vi "Get Steering Frame Velocity from Single Wheel.vi"(4 "acquired wheel states":T2[](array[typedef]), 6 "get motor data":bool, 7 "index info":T1, 8 "error in (no error)":errorcluster, 9 "velocity transform vector in":dbl[](array[numeric]), 10 "velocity transform matrix in":T3, 11 "steering frame in":refnum<class "NI_Robotics_Steering Frame.lvclass">) -> (0 "error out":errorcluster, 1 "velocity transform vector out":dbl[](array[numeric]), 2 "velocity transform matrix out":T3, 3 "steering frame out":refnum<class "NI_Robotics_Steering Frame.lvclass">)   [LabVIEW 2017, in "NI_Robotics_Steering Frame.lvclass"]
uses:
  <vilib>/robotics/Steering/Steering Frame/NI_Robotics_Steering Frame.lvclass
  <vilib>/Analysis/Matrix/Datatypes/RealMatrix.ctl
  <vilib>/robotics/Steering/Wheel/Wheel State.ctl
  <vilib>/robotics/Steering/Steering Frame/NI_Robotics_Steering Frame.lvclass/NI_Robotics_Steering Frame.ctl
  <vilib>/robotics/Steering/Wheel/NI_Robotics_Wheel.lvclass
  <vilib>/Analysis/Matrix/NI_Matrix.lvlib
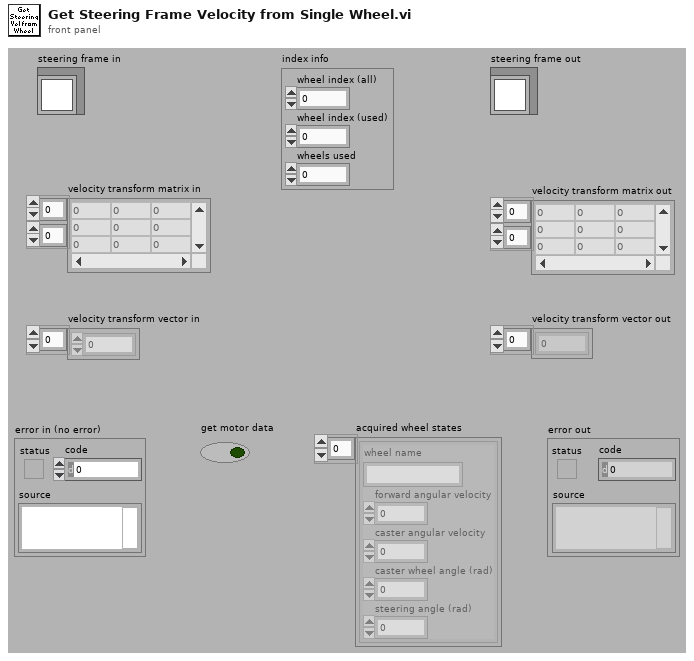
[diagram p1: front panel]
types:
  T1 = cluster{"wheel index (all)":i32, "wheel index (used)":i32, "wheels used":i32}
  T2 = typedef "NI_Robotics_Wheel.lvclass/Wheel State.ctl" = cluster{"wheel name":string, "forward angular velocity":dbl, "caster angular velocity":dbl, "caster wheel angle (rad)":dbl, "steering angle (rad)":dbl}
  T3 = typedef "NI_Matrix.lvlib/RealMatrix.ctl" = dbl[][]
  T4 = typedef "NI_Robotics_Steering Frame.lvclass/Wheel Orientation.ctl" = cluster{"wheel":refnum<class "NI_Robotics_Wheel.lvclass">, "x position":dbl, "y position":dbl, "frame angle (rad)":dbl}
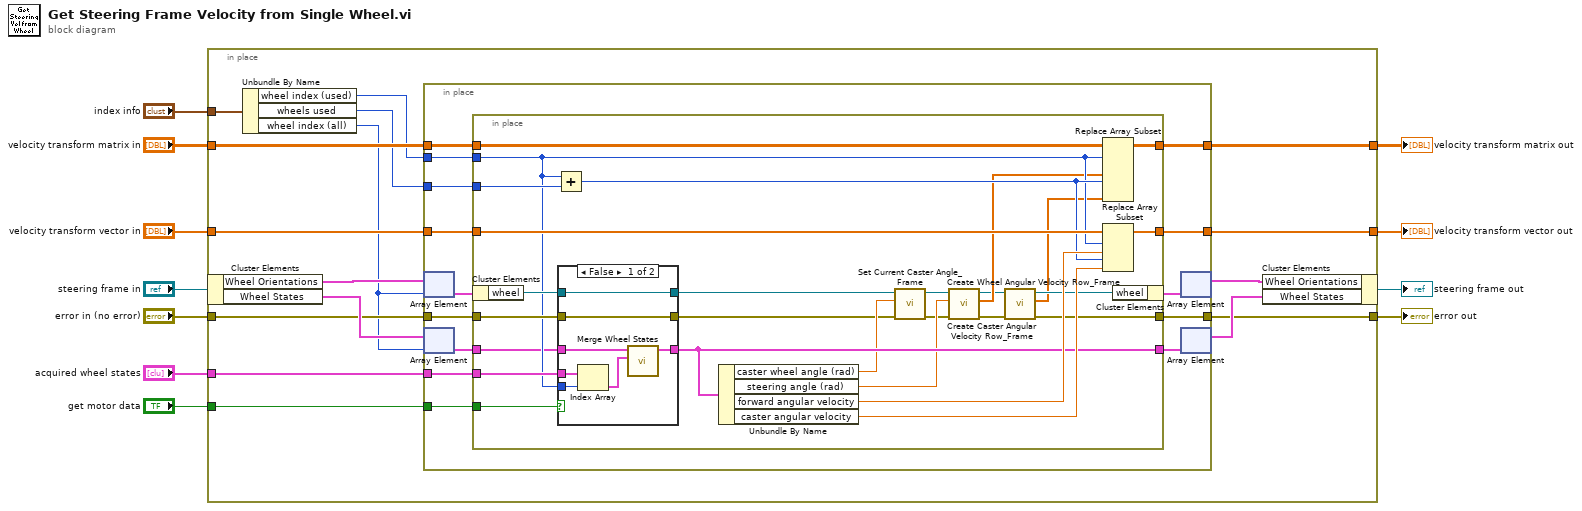
[diagram p0: block diagram]
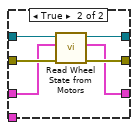
[diagram p2: hidden frame]
diagram:
  n1 = in-place {
    in-place-border: "error in (no error)" -> [w23]
    in-place-border: [w22] -> w8
    in-place-border: "velocity transform matrix in" -> [w21]
    in-place-border: "velocity transform vector in" -> [w20]
    in-place-border: "get motor data" -> [w19]
    in-place-border: "acquired wheel states" -> [w18]
    in-place-border: [w17] -> w3
    in-place-border: [w16] -> w2
    in-place-border: "index info" -> [w15]
    n2 = in-place-cluster #1("steering frame in") -> ("Wheel Orientations"=w27:T4[], "Wheel States"=w25:T2[])
    n3 = Unbundle By Name(w15) -> ("wheel index (used)"=w14:i32, "wheels used"=w13:i32, "wheel index (all)"=w12:i32)
    n4 = in-place {
      in-place-border: [w41] -> w22
      in-place-border: w23 -> [w40]
      in-place-border: w19 -> [w39]
      in-place-border: w20 -> [w38]
      in-place-border: [w37] -> w16
      in-place-border: w21 -> [w36]
      in-place-border: [w35] -> w17
      in-place-border: w13 -> [w34]
      in-place-border: w14 -> [w33]
      in-place-border: w18 -> [w32]
      n5 = in-place-array #2(w27, w12) -> (w31:T4)
      n6 = in-place-array #3(w25, w12) -> (w29:T2)
      n7 = in-place {
        in-place-border: [w47] -> w41
        in-place-border: w40 -> [w67]
        in-place-border: w29 -> [w55]
        in-place-border: w39 -> [w58]
        in-place-border: [w54] -> w28
        in-place-border: w38 -> [w66]
        in-place-border: [w65] -> w37
        in-place-border: w36 -> [w62]
        in-place-border: [w61] -> w35
        in-place-border: w34 -> [w60]
        in-place-border: w33 -> [w56]
        in-place-border: w32 -> [w57]
        n8 = in-place-cluster #4(w31) -> ("wheel"=w68:refnum<class "NI_Robotics_Wheel.lvclass">)
        n9 = Add(x=w56, y=w60) -> (x+y=w59:i32)
        n10 = case shown="False" w58 {
          tunnel: w68 -> [w75 w81]
          tunnel: w67 -> [w73 w80]
          tunnel: [w73 w79] -> w42
          tunnel: [w75 w78] -> w45
          tunnel: [w72 w77] -> w54
          tunnel: w55 -> [w74 w76]
          tunnel: w57 -> [w71 _]
          tunnel: w56 -> [w69 _]
          frame False {
            n11 = Index Array(array=w71, index=w69) -> (element=w70:T2)
            n12 = call <vilib>:"Merge Wheel States.vi"("wheel state with data"=w70, "wheel state with name"=w74) -> ("merged wheel state"=w72:T2)  [unwired: 9 in]
          }
          frame True {
            n13 = call <vilib>:"Read Wheel State from Motors.vi"("error in (no error)"=w80, "wheel state in"=w76, "wheel in"=w81) -> ("error out"=w79:errorcluster, "wheel state out"=w77:T2, "wheel out"=w78:refnum<class "NI_Robotics_Wheel.lvclass">)  [unwired: 6 in]
          }
        }
        n14 = Unbundle By Name(w54) -> ("caster wheel angle (rad)"=w46:dbl, "steering angle (rad)"=w52:dbl, "forward angular velocity"=w64:dbl, "caster angular velocity"=w63:dbl)
        n15 = call <vilib>:"Set Current Caster Angle_Frame.vi"("error in (no error)"=w42, "current caster angle (rad)"=w46, "wheel in"=w45) -> ("error out"=w43:errorcluster, "wheel out"=w44:refnum<class "NI_Robotics_Wheel.lvclass">)  [unwired: 7 in]
        n16 = call <vilib>:"Create Wheel Angular Velocity Row_Frame.vi"("error in (no error)"=w43, "steering angle (rad)"=w52, "wheel in"=w44) -> ("error out"=w48:errorcluster, "wheel angular velocity row"=w53:dbl[], "wheel out"=w51:refnum<class "NI_Robotics_Wheel.lvclass">)  [unwired: 6 in]
        n17 = call <vilib>:"Create Caster Angular Velocity Row_Frame.vi"("error in (no error)"=w48, "wheel in"=w51) -> ("error out"=w47:errorcluster, "wheel caster angular velocity row"=w49:dbl[], "wheel out"=w50:refnum<class "NI_Robotics_Wheel.lvclass">)  [unwired: 6 in, 1 out]
        n18 = Replace Array Subset(array=w62, new element #1=w53, index (row) #1=w56, new element #2=w49, index (row) #2=w59) -> (w61:T3)  [unwired: 2 in]
        n19 = Replace Array Subset(array=w66, new element #1=w64, index #1=w56, new element #2=w63, index #2=w59) -> (w65:dbl[])
        n20 = in-place-cluster #4("wheel"=w50) -> (w30:T4)
      }
      n21 = in-place-array #2(w30) -> (w26:T4[])  [unwired: 1 out]
      n22 = in-place-array #3(w28) -> (w24:T2[])  [unwired: 1 out]
    }
    n23 = in-place-cluster #1("Wheel Orientations"=w26, "Wheel States"=w24) -> (→"steering frame out":refnum<class "NI_Robotics_Steering Frame.lvclass">)
  }
  "error out" <- w8
  "velocity transform matrix out" <- w3
  "velocity transform vector out" <- w2
